vi "Open Excel.vi"() -> ()   [LabVIEW 2014]
uses:
  <vilib>/addons/_office/excel.llb/Excel Get Data ([str]).vi
  <vilib>/addons/_office/NI_ReportGenerationToolkit.lvlib
  <vilib>/Utility/NIReport.llb/NI_report.lvclass
  <vilib>/Utility/NIReport.llb/Excel/NI_Excel.lvclass
panel:
  in  "template (empty)":path
  out "data":string[][](array[string])
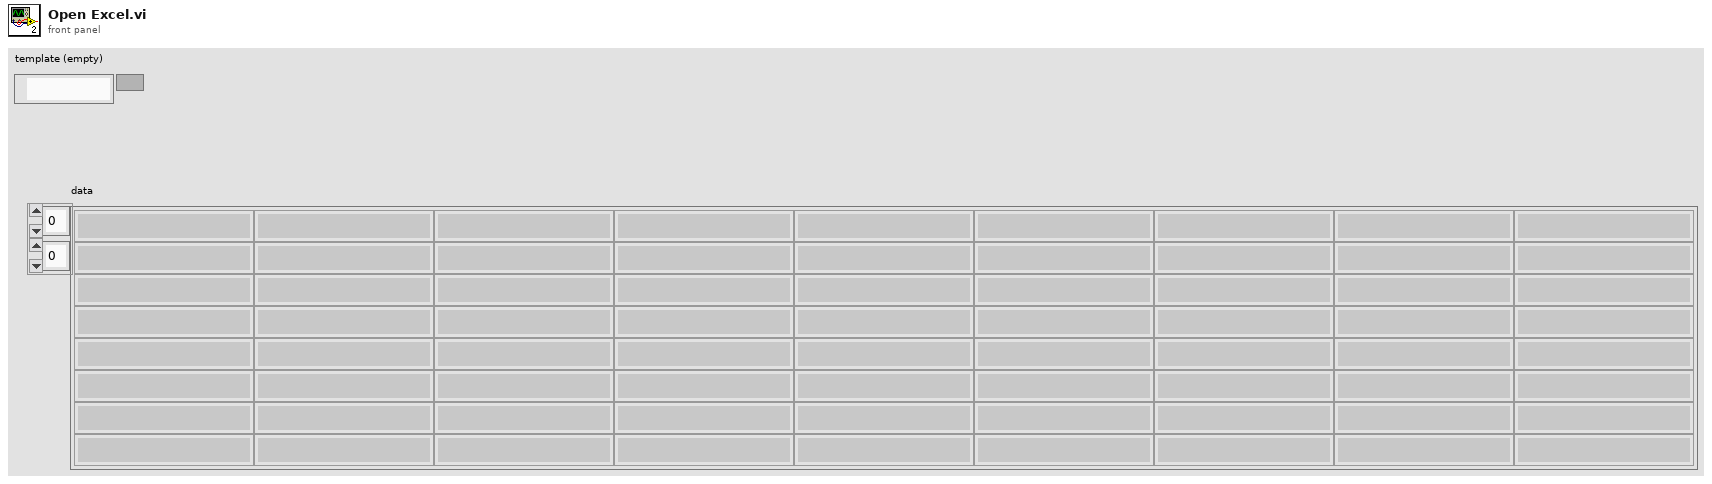
[diagram p1: front panel]
types:
  T1 = enum16{"maximized", "minimized", "normal", "no change"}
  T2 = enum16{"Standard Report", "HTML", "Word", "Excel"}
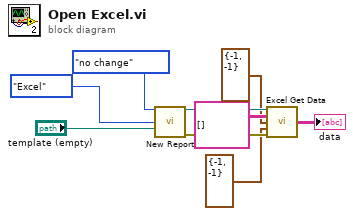
[diagram p0: block diagram]
diagram:
  n1 = call <vilib>:"New Report.vi"("window state (normal)"=T1."no change", "report type"=T2."Excel", "template (empty)"="template (empty)") -> ("report out"=w9:refnum<class "NI_report.lvclass">, "error out"=w8:errorcluster)  [unwired: 11 in]
  n2 = call-poly <vilib>:"Excel Get Data.vi"("report in"=w9, "data type"=string[][] [], "start (-1, -1)"=cluster{"row":i32, "column":i32} {"row"=-1, "column"=-1}, "end (-1, -1)"=cluster{"row":i32, "column":i32} {"row"=-1, "column"=-1}, "error in (no error)"=w8) -> ("data"=→"data":string[][])  [unwired: 8 in, 2 out]
